vi "tm_stopcapture.vi"(8 "error in (no error)":errorcluster, 11 "Handle in":u32) -> (0 "error out":errorcluster, 3 "Handle out":u32)   [LabVIEW 2015]
uses:
  tmcamcon.dll
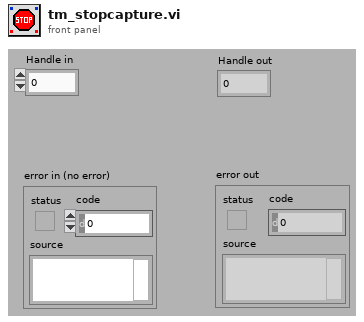
[diagram p1: front panel]
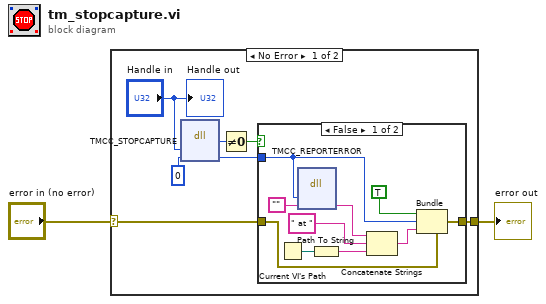
[diagram p0: block diagram]
diagram:
  n1 = case shown="No Error" "error in (no error)" {
    selector: "error in (no error)" -> [w5 w21]
    tunnel: [w4 w21] -> w1
    frame No Error {
      n2 = dll-call lib="tmcamcon.dll" fn="TMCC_STOPCAPTURE"("index"="Handle in", "Erval"=0) -> (w9:u32, "Erval"=w6:i32)  [unwired: 4 in, 2 out]
      n3 = Not Equal To 0?(x=w9) -> (x != 0?=w7:bool)
      n4 = case shown="False" w7 {
        tunnel: w5 -> [w19 w20]
        tunnel: [w18 w20] -> w4
        tunnel: w6 -> [w12 _]
        frame False {
          n5 = Current VI's Path() -> (path=w17:path)
          n6 = dll-call lib="tmcamcon.dll" fn="TMCC_REPORTERROR"("error"=w12, "buf"="") -> ("buf"=w11:string)  [unwired: 5 in, 2 out]
          n7 = Path To String(path=w17) -> (string=w13:string)
          n8 = Concatenate Strings(w11, " at ", w13) -> (w16:string)
          n9 = Bundle(cluster=w19, "status"=TRUE, "code"=w12, "source"=w16) -> (w18:errorcluster)
        }
        frame True {
        }
      }
      "Handle out" <- "Handle in"
    }
    frame Error {
    }
  }
  "error out" <- w1
